vi "Write MERCANCIA.vi"(8 "error in (no error)":errorcluster, 10 "MERCANCIA":refnum<vi>, 11 "BD_CAFE_USD_ING in":refnum<class "BD_CAFE_USD_ING.lvclass">) -> (0 "error out":errorcluster, 3 "BD_CAFE_USD_ING out":refnum<class "BD_CAFE_USD_ING.lvclass">)   [LabVIEW 2019, in "BD_CAFE_USD_ING.lvlib" / "BD_CAFE_USD_ING.lvclass"]
uses:
  BD_CAFE_USD_ING.lvclass
  BD_CAFE_USD_ING.lvclass/BD_CAFE_USD_ING.ctl
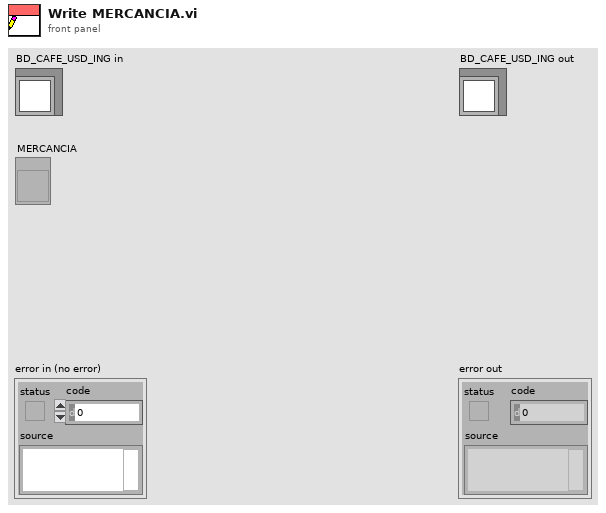
[diagram p1: front panel]
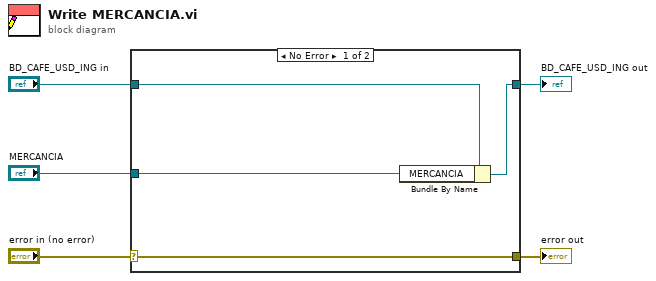
[diagram p0: block diagram]
diagram:
  n1 = case shown="No Error" "error in (no error)" {
    selector: "error in (no error)" -> [w9 w10]
    tunnel: [w9 w10] -> w4
    tunnel: [w7 w11] -> w2
    tunnel: "BD_CAFE_USD_ING in" -> [w8 w11]
    tunnel: "MERCANCIA" -> [w6 _]
    frame No Error {
      n2 = Bundle By Name(cluster=w8, "MERCANCIA"=w6) -> (w7:refnum<class "BD_CAFE_USD_ING.lvclass">)
    }
    frame Error {
    }
  }
  "error out" <- w4
  "BD_CAFE_USD_ING out" <- w2
